vi "Device Enumeration Path.vi"() -> (3 "Device Enumeration Path":path)   [LabVIEW 2020, in "HAL Config.lvlib" / "HAL Editor.lvclass"]
uses:
  HAL Editor.lvclass
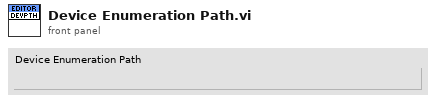
[diagram p1: front panel]
types:
  T1 = enum32{"invalid app kind", "Development System", "Run Time System", "Student Edition", "Embedded LabVIEW", "Evaluation", "Custom", "Community Edition"}
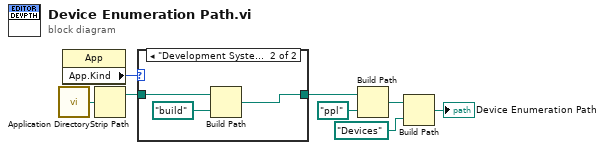
[diagram p0: block diagram]
diagram:
  n1 = call <vilib>:"Application Directory.vi"() -> ("Application Directory"=w7:path)
  n2 = property class="App"() -> ("App.Kind"=w8:T1)  [unwired: 2 in, 2 out]
  n3 = Strip Path(path=w7) -> (stripped path=w6:path)  [unwired: 1 out]
  n4 = case shown="\"Development System\"" w8 {
    tunnel: [w9 w11] -> w5
    tunnel: w6 -> [w9 w10]
    frame Default {
    }
    frame "Development System" {
      n5 = Build Path(base path=w10, name or relative path=path "build") -> (appended path=w11:path)
    }
  }
  n6 = Build Path(base path=w5, name or relative path=path "ppl") -> (appended path=w3:path)
  n7 = Build Path(base path=w3, name or relative path=path "Devices") -> (appended path=→"Device Enumeration Path":path)
